vi "GeoData.vi"() -> ()   [LabVIEW 2017] (continued)
County\tH1\n71933\t5097\tBonnerdale\tAR\tMontgomery County\tH1\n71961\t5097\tOden\tAR\tMontgomery County\tH1\n71943\t5097\tGlenwood\tAR\tMontgomery County\tH1\n71969\t5097\tSims\tAR\tMontgomery County\tH1\n71965\t5097\tPencil bluff\tAR\tMontgomery County\tH1\n71970\t5097\tStory\tAR\tMontgomery County\tH1\n71960\t5097\tNorman\tAR\tMontgomery County\tH1\n71957\t5097\tMount ida\tAR\tMontgomery County\tH1\n71949\t5097\tJessieville\tAR\tMontgomery County\tH1\n71935\t5097\tCaddo gap\tAR\tMontgomery County\tH1\n71858\t5099\tRosston\tAR\tNevada County\tH1\n71764\t5099\tStephens\tAR\tNevada County\tH1\n71827\t5099\tBuckner\tAR\tNevada County\tH1\n71770\t5099\tWaldo\tAR\tNevada County\tH1\n71857\t5099\tPrescott\tAR\tNevada County\tH1\n71828\t5099\tCale\tAR\tNevada County\tH1\n71752\t5099\tMc neil\tAR\tNevada County\tH1\n71722\t5099\tBluff city\tAR\tNevada County\tH1\n71835\t5099\tEmmet\tAR\tNevada County\tH1\n71864\t5099\tWillisville\tAR\tNevada County\tH1\n71860\t5099\tStamps\tAR\tNevada County\tH1\n72628\t5101\tDeer\tAR\tNewton County\tH1\n72685\t5101\tWestern grove\tAR\tNewton County\tH1\n72641\t5101\tJasper\tAR\tNewton County\tH1\n72670\t5101\tPonca\tAR\tNewton County\tH1\n72601\t5101\tHarrison\tAR\tNewton County\tH1\n72624\t5101\tCompton\tAR\tNewton County\tH1\n72638\t5101\tGreen forest\tAR\tNewton County\tH1\n72683\t5101\tVendor\tAR\tNewton County\tH1\n72742\t5101\tKingston\tAR\tNewton County\tH1\n72666\t5101\tParthenon\tAR\tNewton County\tH1\n72640\t5101\tHasty\tAR\tNewton County\tH1\n72655\t5101\tMount judea\tAR\tNewton County\tH1\n72648\t5101\tMarble falls\tAR\tNewton County\tH1\n71701\t5103\tCamden\tAR\tOuachita County\tH1\n71764\t5103\tStephens\tAR\tOuachita County\tH1\n71720\t5103\tBearden\tAR\tOuachita County\tH1\n71763\t5103\tSparkman\tAR\tOuachita County\tH1\n71751\t5103\tLouann\tAR\tOuachita County\tH1\n71857\t5103\tPrescott\tAR\tOuachita County\tH1\n71762\t5103\tSmackover\tAR\tOuachita County\tH1\n71726\t5103\tChidester\tAR\tOuachita County\tH1\n72001\t5105\tAdona\tAR\tPerry County\tH1\n72857\t5105\tPlainview\tAR\tPerry County\tH1\n72126\t5105\tPerryville\tAR\tPerry County\tH1\n72135\t5105\tRoland\tAR\tPerry County\tH1\n72853\t5105\tOla\tAR\tPerry County\tH1\n72125\t5105\tPerry\tAR\tPerry County\tH1\n72034\t5105\tConway\tAR\tPerry County\tH1\n72025\t5105\tCasa\tAR\tPerry County\tH1\n72070\t5105\tHouston\tAR\tPerry County\tH1\n72016\t5105\tBigelow\tAR\tPerry County\tH1\n72366\t5107\tMarvell\tAR\tPhillips County\tH1\n72355\t5107\tLexa\tAR\tPhillips County\tH1\n72312\t5107\tBarton\tAR\tPhillips County\tH1\n72328\t5107\tCrumrod\tAR\tPhillips County\tH1\n72383\t5107\tTurner\tAR\tPhillips County\tH1\n72353\t5107\tLambrook\tAR\tPhillips County\tH1\n72342\t5107\tHelena\tAR\tPhillips County\tH1\n72374\t5107\tPoplar grove\tAR\tPhillips County\tH1\n72389\t5107\tWabash\tAR\tPhillips County\tH1\n72390\t5107\tWest helena\tAR\tPhillips County\tH1\n72369\t5107\tOneida\tAR\tPhillips County\tH1\n72333\t5107\tElaine\tAR\tPhillips County\tH1\n72367\t5107\tMellwood\tAR\tPhillips County\tH1\n72069\t5107\tHolly grove\tAR\tPhillips County\tH1\n71971\t5109\tUmpire\tAR\tPike County\tH1\n71943\t5109\tGlenwood\tAR\tPike County\tH1\n71922\t5109\tAntoine\tAR\tPike County\tH1\n71921\t5109\tAmity\tAR\tPike County\tH1\n71958\t5109\tMurfreesboro\tAR\tPike County\tH1\n71959\t5109\tNewhope\tAR\tPike County\tH1\n71952\t5109\tLangley\tAR\tPike County\tH1\n71852\t5109\tNashville\tAR\tPike County\tH1\n71935\t5109\tCaddo gap\tAR\tPike County\tH1\n71940\t5109\tDelight\tAR\tPike County\tH1\n71950\t5109\tKirby\tAR\tPike County\tH1\n72421\t5111\tCash\tAR\tPoinsett County\tH1\n72429\t5111\tFisher\tAR\tPoinsett County\tH1\n72475\t5111\tWaldenburg\tAR\tPoinsett County\tH1\n72472\t5111\tTrumann\tAR\tPoinsett County\tH1\n72354\t5111\tLepanto\tAR\tPoinsett County\tH1\n72432\t5111\tHarrisburg\tAR\tPoinsett County\tH1\n72386\t5111\tTyronza\tAR\tPoinsett County\tH1\n72419\t5111\tCaraway\tAR\tPoinsett County\tH1\n72365\t5111\tMarked tree\tAR\tPoinsett County\tH1\n72324\t5111\tCherry valley\tAR\tPoinsett County\tH1\n72377\t5111\tRivervale\tAR\tPoinsett County\tH1\n72479\t5111\tWeiner\tAR\tPoinsett County\tH1\n71944\t5113\tGrannis\tAR\tPolk County\tH1\n71945\t5113\tHatfield\tAR\tPolk County\tH1\n71961\t5113\tOden\tAR\tPolk County\tH1\n71937\t5113\tCove\tAR\tPolk County\tH1\n71841\t5113\tGillham\tAR\tPolk County\tH1\n71953\t5113\tMena\tAR\tPolk County\tH1\n71973\t5113\tWickes\tAR\tPolk County\tH1\n71972\t5113\tVandervoort\tAR\tPolk County\tH1\n71932\t5113\tBoard camp\tAR\tPolk County\tH1\n72801\t5115\tRussellville\tAR\tPope County\tH1\n72686\t5115\tWitts springs\tAR\tPope County\tH1\n72856\t5115\tPelsor\tAR\tPope County\tH1\n72802\t5115\tRussellville\tAR\tPope County\tH1\n72823\t5115\tAtkins\tAR\tPope County\tH1\n72843\t5115\tHector\tAR\tPope County\tH1\n72858\t5115\tPottsville\tAR\tPope County\tH1\n72847\t5115\tLondon\tAR\tPope County\tH1\n72811\t5115\tRussellville\tAR\tPope County\tH1\n72080\t5115\tJerusalem\tAR\tPope County\tH1\n72063\t5115\tHattieville\tAR\tPope County\tH1\n72846\t5115\tLamar\tAR\tPope County\tH1\n72837\t5115\tDover\tAR\tPope County\tH1\n72812\t5115\tRussellville\tAR\tPope County\tH1\n72679\t5115\tTilly\tAR\tPope County\tH1\n72170\t5117\tUlm\tAR\tPrairie County\tH1\n72134\t5117\tRoe\tAR\tPrairie County\tH1\n72086\t5117\tLonoke\tAR\tPrairie County\tH1\n72041\t5117\tDe valls bluff\tAR\tPrairie County\tH1\n72066\t5117\tHickory plains\tAR\tPrairie County\tH1\n72040\t5117\tDes arc\tAR\tPrairie County\tH1\n72060\t5117\tGriffithville\tAR\tPrairie County\tH1\n72160\t5117\tStuttgart\tAR\tPrairie County\tH1\n72024\t5117\tCarlisle\tAR\tPrairie County\tH1\n72017\t5117\tBiscoe\tAR\tPrairie County\tH1\n72176\t5117\tWard\tAR\tPrairie County\tH1\n72064\t5117\tHazen\tAR\tPrairie County\tH1\n72116\t5119\tNorth little rock\tAR\tPulaski County\tH1\n72205\t5119\tLittle rock\tAR\tPulaski County\tH1\n72223\t5119\tLittle rock\tAR\tPulaski County\tH1\n72204\t5119\tLittle rock\tAR\tPulaski County\tH1\n72207\t5119\tLittle rock\tAR\tPulaski County\tH1\n72227\t5119\tLittle rock\tAR\tPulaski County\tH1\n72078\t5119\tJacksonville\tAR\tPulaski County\tH1\n72199\t5119\tNorth little rock\tAR\tPulaski County\tH1\n72065\t5119\tHensley\tAR\tPulaski County\tH1\n72002\t5119\tAlexander\tAR\tPulaski County\tH1\n72209\t5119\tLittle rock\tAR\tPulaski County\tH1\n72126\t5119\tPerryville\tAR\tPulaski County\tH1\n72115\t5119\tNorth little rock\tAR\tPulaski County\tH1\n72255\t5119\tLittle rock\tAR\tPulaski County\tH1\n72023\t5119\tCabot\tAR\tPulaski County\tH1\n72120\t5119\tSherwood\tAR\tPulaski County\tH1\n72135\t5119\tRoland\tAR\tPulaski County\tH1\n72217\t5119\tLittle rock\tAR\tPulaski County\tH1\n72099\t5119\tLittle rock air force base\tAR\tPulaski County\tH1\n72046\t5119\tEngland\tAR\tPulaski County\tH1\n72113\t5119\tMaumelle\tAR\tPulaski County\tH1\n72202\t5119\tLittle rock\tAR\tPulaski County\tH1\n72214\t5119\tLittle rock\tAR\tPulaski County\tH1\n72117\t5119\tNorth little rock\tAR\tPulaski County\tH1\n72142\t5119\tScott\tAR\tPulaski County\tH1\n72190\t5119\tNorth little rock\tAR\tPulaski County\tH1\n72106\t5119\tMayflower\tAR\tPulaski County\tH1\n72053\t5119\tCollege station\tAR\tPulaski County\tH1\n72076\t5119\tJacksonville\tAR\tPulaski County\tH1\n72210\t5119\tLittle rock\tAR\tPulaski County\tH1\n72211\t5119\tLittle rock\tAR\tPulaski County\tH1\n72206\t5119\tLittle rock\tAR\tPulaski County\tH1\n72216\t5119\tLittle rock\tAR\tPulaski County\tH1\n72225\t5119\tLittle rock\tAR\tPulaski County\tH1\n72124\t5119\tNorth little rock\tAR\tPulaski County\tH1\n72173\t5119\tVilonia\tAR\tPulaski County\tH1\n72215\t5119\tLittle rock\tAR\tPulaski County\tH1\n72203\t5119\tLittle rock\tAR\tPulaski County\tH1\n72219\t5119\tLittle rock\tAR\tPulaski County\tH1\n72260\t5119\tLittle rock\tAR\tPulaski County\tH1\n72103\t5119\tMabelvale\tAR\tPulaski County\tH1\n72016\t5119\tBigelow\tAR\tPulaski County\tH1\n72132\t5119\tRedfield\tAR\tPulaski County\tH1\n72222\t5119\tLittle rock\tAR\tPulaski County\tH1\n72119\t5119\tNorth little rock\tAR\tPulaski County\tH1\n72180\t5119\tWoodson\tAR\tPulaski County\tH1\n72114\t5119\tNorth little rock\tAR\tPulaski County\tH1\n72201\t5119\tLittle rock\tAR\tPulaski County\tH1\n72212\t5119\tLittle rock\tAR\tPulaski County\tH1\n72118\t5119\tNorth little rock\tAR\tPulaski County\tH1\n72122\t5119\tParon\tAR\tPulaski County\tH1\n72221\t5119\tLittle rock\tAR\tPulaski County\tH1\n72231\t5119\tLittle rock\tAR\tPulaski County\tH1\n72183\t5119\tWrightsville\tAR\tPulaski County\tH1\n72164\t5119\tSweet home\tAR\tPulaski County\tH1\n72413\t5121\tBiggers\tAR\tRandolph County\tH1\n72449\t5121\tO kean\tAR\tRandolph County\tH1\n72455\t5121\tPocahontas\tAR\tRandolph County\tH1\n72554\t5121\tMammoth spring\tAR\tRandolph County\tH1\n72459\t5121\tRavenden\tAR\tRandolph County\tH1\n72462\t5121\tReyno\tAR\tRandolph County\tH1\n72476\t5121\tWalnut ridge\tAR\tRandolph County\tH1\n72460\t5121\tRavenden springs\tAR\tRandolph County\tH1\n72434\t5121\tImboden\tAR\tRandolph County\tH1\n72444\t5121\tMaynard\tAR\tRandolph County\tH1\n72478\t5121\tWarm springs\tAR\tRandolph County\tH1\n72422\t5121\tCorning\tAR\tRandolph County\tH1\n72425\t5121\tDelaplaine\tAR\tRandolph County\tH1\n72021\t5123\tBrinkley\tAR\tSt. Francis County\tH1\n72396\t5123\tWynne\tAR\tSt. Francis County\tH1\n72360\t5123\tMarianna\tAR\tSt. Francis County\tH1\n72346\t5123\tHeth\tAR\tSt. Francis County\tH1\n72392\t5123\tWheatley\tAR\tSt. Francis County\tH1\n72335\t5123\tForrest city\tAR\tSt. Francis County\tH1\n72348\t5123\tHughes\tAR\tSt. Francis County\tH1\n72326\t5123\tColt\tAR\tSt. Francis County\tH1\n72340\t5123\tGoodwin\tAR\tSt. Francis County\tH1\n72376\t5123\tProctor\tAR\tSt. Francis County\tH1\n72394\t5123\tWidener\tAR\tSt. Francis County\tH1\n72372\t5123\tPalestine\tAR\tSt. Francis County\tH1\n72359\t5123\tMadison\tAR\tSt. Francis County\tH1\n72322\t5123\tCaldwell\tAR\tSt. Francis County\tH1\n72019\t5125\tBenton\tAR\tSaline County\tH1\n72018\t5125\tBenton\tAR\tSaline County\tH1\n72065\t5125\tHensley\tAR\tSaline County\tH1\n72002\t5125\tAlexander\tAR\tSaline County\tH1\n72104\t5125\tMalvern\tAR\tSaline County\tH1\n72167\t5125\tTraskwood\tAR\tSaline County\tH1\n72022\t5125\tBryant\tAR\tSaline County\tH1\n72210\t5125\tLittle rock\tAR\tSaline County\tH1\n72206\t5125\tLittle rock\tAR\tSaline County\tH1\n72089\t5125\tBryant\tAR\tSaline County\tH1\n71909\t5125\tHot springs village\tAR\tSaline County\tH1\n72087\t5125\tLonsdale\tAR\tSaline County\tH1\n72015\t5125\tBenton\tAR\tSaline County\tH1\n72103\t5125\tMabelvale\tAR\tSaline County\tH1\n72011\t5125\tBauxite\tAR\tSaline County\tH1\n72122\t5125\tParon\tAR\tSaline County\tH1\n72944\t5127\tMansfield\tAR\tScott County\tH1\n72950\t5127\tParks\tAR\tScott County\tH1\n71953\t5127\tMena\tAR\tScott County\tH1\n72927\t5127\tBooneville\tAR\tScott County\tH1\n72841\t5127\tHarvey\tAR\tScott County\tH1\n72958\t5127\tWaldron\tAR\tScott County\tH1\n72926\t5127\tBoles\tAR\tScott County\tH1\n72838\t5127\tGravelly\tAR\tScott County\tH1\n72833\t5127\tDanville\tAR\tScott County\tH1\n72686\t5129\tWitts springs\tAR\tSearcy County\tH1\n72617\t5129\tBig flat\tAR\tSearcy County\tH1\n72636\t5129\tGilbert\tAR\tSearcy County\tH1\n72680\t5129\tTimbo\tAR\tSearcy County\tH1\n72685\t5129\tWestern grove\tAR\tSearcy County\tH1\n72650\t5129\tMarshall\tAR\tSearcy County\tH1\n72639\t5129\tHarriet\tAR\tSearcy County\tH1\n72629\t5129\tDennard\tAR\tSearcy County\tH1\n72675\t5129\tSaint joe\tAR\tSearcy County\tH1\n72633\t5129\tEverton\tAR\tSearcy County\tH1\n72645\t5129\tLeslie\tAR\tSearcy County\tH1\n72669\t5129\tPindall\tAR\tSearcy County\tH1\n72687\t5129\tYellville\tAR\tSearcy County\tH1\n72679\t5129\tTilly\tAR\tSearcy County\tH1\n72903\t5131\tFort smith\tAR\tSebastian County\tH1\n72933\t5131\tCharleston\tAR\tSebastian County\tH1\n72944\t5131\tMansfield\tAR\tSebastian County\tH1\n72918\t5131\tFort smith\tAR\tSebastian County\tH1\n72919\t5131\tFort smith\tAR\tSebastian County\tH1\n72936\t5131\tGreenwood\tAR\tSebastian County\tH1\n72916\t5131\tFort smith\tAR\tSebastian County\tH1\n72905\t5131\tFort smith\tAR\tSebastian County\tH1\n72904\t5131\tFort smith\tAR\tSebastian County\tH1\n72927\t5131\tBooneville\tAR\tSebastian County\tH1\n72938\t5131\tHartford\tAR\tSebastian County\tH1\n72940\t5131\tHuntington\tAR\tSebastian County\tH1\n72941\t5131\tLavaca\tAR\tSebastian County\tH1\n72908\t5131\tFort smith\tAR\tSebastian County\tH1\n72930\t5131\tCecil\tAR\tSebastian County\tH1\n72914\t5131\tFort smith\tAR\tSebastian County\tH1\n72913\t5131\tFort smith\tAR\tSebastian County\tH1\n72923\t5131\tBarling\tAR\tSebastian County\tH1\n72937\t5131\tHackett\tAR\tSebastian County\tH1\n72902\t5131\tFort smith\tAR\tSebastian County\tH1\n72917\t5131\tFort smith\tAR\tSebastian County\tH1\n72945\t5131\tMidland\tAR\tSebastian County\tH1\n72901\t5131\tFort smith\tAR\tSebastian County\tH1\n72906\t5131\tFort smith\tAR\tSebastian County\tH1\n71832\t5133\tDe queen\tAR\tSevier County\tH1\n71841\t5133\tGillham\tAR\tSevier County\tH1\n71833\t5133\tDierks\tAR\tSevier County\tH1\n71842\t5133\tHoratio\tAR\tSevier County\tH1\n71846\t5133\tLockesburg\tAR\tSevier County\tH1\n71823\t5133\tBen lomond\tAR\tSevier County\tH1\n72542\t5135\tHardy\tAR\tSharp County\tH1\n72469\t5135\tStrawberry\tAR\tSharp County\tH1\n72466\t5135\tSmithville\tAR\tSharp County\tH1\n72554\t5135\tMammoth spring\tAR\tSharp County\tH1\n72521\t5135\tCave city\tAR\tSharp County\tH1\n72529\t5135\tCherokee village\tAR\tSharp County\tH1\n72459\t5135\tRavenden\tAR\tSharp County\tH1\n72532\t5135\tEvening shade\tAR\tSharp County\tH1\n72579\t5135\tSulphur rock\tAR\tSharp County\tH1\n72482\t5135\tWilliford\tAR\tSharp County\tH1\n72513\t5135\tAsh flat\tAR\tSharp County\tH1\n72569\t5135\tPoughkeepsie\tAR\tSharp County\tH1\n72577\t5135\tSidney\tAR\tSharp County\tH1\n72153\t5137\tShirley\tAR\tStone County\tH1\n72044\t5137\tEdgemont\tAR\tStone County\tH1\n72051\t5137\tFox\tAR\tStone County\tH1\n72617\t5137\tBig flat\tAR\tStone County\tH1\n72567\t5137\tPleasant grove\tAR\tStone County\tH1\n72680\t5137\tTimbo\tAR\tStone County\tH1\n72556\t5137\tMelbourne\tAR\tStone County\tH1\n72530\t5137\tDrasco\tAR\tStone County\tH1\n72650\t5137\tMarshall\tAR\tStone County\tH1\n72550\t5137\tLocust grove\tAR\tStone County\tH1\n72540\t5137\tGuion\tAR\tStone County\tH1\n72555\t5137\tMarcella\tAR\tStone County\tH1\n72645\t5137\tLeslie\tAR\tStone County\tH1\n72657\t5137\tTimbo\tAR\tStone County\tH1\n72031\t5137\tClinton\tAR\tStone County\tH1\n72519\t5137\tCalico rock\tAR\tStone County\tH1\n72533\t5137\tFifty six\tAR\tStone County\tH1\n72560\t5137\tMountain view\tAR\tStone County\tH1\n72663\t5137\tOnia\tAR\tStone County\tH1\n71730\t5139\tEl dorado\tAR\tUnion County\tH1\n71747\t5139\tHuttig\tAR\tUnion County\tH1\n71750\t5139\tLawson\tAR\tUnion County\tH1\n71764\t5139\tStephens\tAR\tUnion County\tH1\n71759\t5139\tNorphlet\tAR\tUnion County\tH1\n71753\t5139\tMagnolia\tAR\tUnion County\tH1\n71762\t5139\tSmackover\tAR\tUnion County\tH1\n71731\t5139\tEl dorado\tAR\tUnion County\tH1\n71724\t5139\tCalion\tAR\tUnion County\tH1\n71765\t5139\tStrong\tAR\tUnion County\tH1\n71749\t5139\tJunction city\tAR\tUnion County\tH1\n71758\t5139\tMount holly\tAR\tUnion County\tH1\n72013\t5141\tBee branch\tAR\tVan Buren County\tH1\n72153\t5141\tShirley\tAR\tVan Buren County\tH1\n72039\t5141\tDamascus\tAR\tVan Buren County\tH1\n72030\t5141\tCleveland\tAR\tVan Buren County\tH1\n72067\t5141\tHigden\tAR\tVan Buren County\tH1\n72131\t5141\tQuitman\tAR\tVan Buren County\tH1\n72028\t5141\tChoctaw\tAR\tVan Buren County\tH1\n72629\t5141\tDennard\tAR\tVan Buren County\tH1\n72080\t5141\tJerusalem\tAR\tVan Buren County\tH1\n72645\t5141\tLeslie\tAR\tVan Buren County\tH1\n72031\t5141\tClinton\tAR\tVan Buren County\tH1\n72088\t5141\tFairfield bay\tAR\tVan Buren County\tH1\n72141\t5141\tScotland\tAR\tVan Buren County\tH1\n72679\t5141\tTilly\tAR\tVan Buren County\tH1\n72703\t5143\tFayetteville\tAR\tWashington County\tH1\n72730\t5143\tFarmington\tAR\tWashington County\tH1\n72773\t5143\tWesley\tAR\tWashington County\tH1\n72765\t5143\tSpringdale\tAR\tWashington County\tH1\n72728\t5143\tElm springs\tAR\tWashington County\tH1\n72761\t5143\tSiloam springs\tAR\tWashington County\tH1\n72764\t5143\tSpringdale\tAR\tWashington County\tH1\n72741\t5143\tJohnson\tAR\tWashington County\tH1\n72770\t5143\tTontitown\tAR\tWashington County\tH1\n72717\t5143\tCanehill\tAR\tWashington County\tH1\n72734\t5143\tGentry\tAR\tWashington County\tH1\n72727\t5143\tElkins\tAR\tWashington County\tH1\n72769\t5143\tSummers\tAR\tWashington County\tH1\n72766\t5143\tSpringdale\tAR\tWashington County\tH1\n72749\t5143\tMorrow\tAR\tWashington County\tH1\n72704\t5143\tFayetteville\tAR\tWashington County\tH1\n72959\t5143\tWinslow\tAR\tWashington County\tH1\n72948\t5143\tNatural dam\tAR\tWashington County\tH1\n72737\t5143\tGreenland\tAR\tWashington County\tH1\n72738\t5143\tHindsville\tAR\tWashington County\tH1\n72729\t5143\tEvansville\tAR\tWashington County\tH1\n72762\t5143\tSpringdale\tAR\tWashington County\tH1\n72774\t5143\tWest fork\tAR\tWashington County\tH1\n72753\t5143\tPrairie grove\tAR\tWashington County\tH1\n72702\t5143\tFayetteville\tAR\tWashington County\tH1\n72744\t5143\tLincoln\tAR\tWashington County\tH1\n72735\t5143\tGoshen\tAR\tWashington County\tH1\n72701\t5143\tFayetteville\tAR\tWashington County\tH1\n72010\t5145\tBald knob\tAR\tWhite County\tH1\n72568\t5145\tPleasant plains\tAR\tWhite County\tH1\n72068\t5145\tHigginson\tAR\tWhite County\tH1\n72178\t5145\tWest point\tAR\tWhite County\tH1\n72139\t5145\tRussell\tAR\tWhite County\tH1\n72012\t5145\tBeebe\tAR\tWhite County\tH1\n72121\t5145\tPangburn\tAR\tWhite County\tH1\n72085\t5145\tLetona\tAR\tWhite County\tH1\n72081\t5145\tJudsonia\tAR\tWhite County\tH1\n72102\t5145\tMc rae\tAR\tWhite County\tH1\n72143\t5145\tSearcy\tAR\tWhite County\tH1\n72052\t5145\tGarner\tAR\tWhite County\tH1\n72082\t5145\tKensett\tAR\tWhite County\tH1\n72045\t5145\tEl paso\tAR\tWhite County\tH1\n72060\t5145\tGriffithville\tAR\tWhite County\tH1\n72149\t5145\tSearcy\tAR\tWhite County\tH1\n72020\t5145\tBradford\tAR\tWhite County\tH1\n72173\t5145\tVilonia\tAR\tWhite County\tH1\n72111\t5145\tMount vernon\tAR\tWhite County\tH1\n72145\t5145\tSearcy\tAR\tWhite County\tH1\n72136\t5145\tRomance\tAR\tWhite County\tH1\n72137\t5145\tRose bud\tAR\tWhite County\tH1\n72112\t5147\tNewport\tAR\tWoodruff County\tH1\n72021\t5147\tBrinkley\tAR\tWoodruff County\tH1\n72396\t5147\tWynne\tAR\tWoodruff County\tH1\n72006\t5147\tAugusta\tAR\tWoodruff County\tH1\n72123\t5147\tPatterson\tAR\tWoodruff County\tH1\n72392\t5147\tWheatley\tAR\tWoodruff County\tH1\n72059\t5147\tGregory\tAR\tWoodruff County\tH1\n72101\t5147\tMc crory\tAR\tWoodruff County\tH1\n72036\t5147\tCotton plant\tAR\tWoodruff County\tH1\n72074\t5147\tHunter\tAR\tWoodruff County\tH1\n72857\t5149\tPlainview\tAR\tYell County\tH1\n72943\t5149\tMagazine\tAR\tYell County\tH1\n72853\t5149\tOla\tAR\tYell County\tH1\n72842\t5149\tHavana\tAR\tYell County\tH1\n72824\t5149\tBelleville\tAR\tYell County\tH1\n72828\t5149\tBriggsville\tAR\tYell County\tH1\n72841\t5149\tHarvey\tAR\tYell County\tH1\n72025\t5149\tCasa\tAR\tYell County\tH1\n72827\t5149\tBluffton\tAR\tYell County\tH1\n72860\t5149\tRover\tAR\tYell County\tH1\n72829\t5149\tCenterville\tAR\tYell County\tH1\n72834\t5149\tDardanelle\tAR\tYell County\tH1\n72838\t5149\tGravelly\tAR\tYell County\tH1\n72833\t5149\tDanville\tAR\tYell County\tH1\n94501\t6001\tAlameda\tCA\tAlameda County\tH1\n94560\t6001\tNewark\tCA\tAlameda County\tH1\n94577\t6001\tSan leandro\tCA\tAlameda County\tH1\n94578\t6001\tSan leandro\tCA\tAlameda County\tH1\n94550\t6001\tLivermore\tCA\tAlameda County\tH1\n94611\t6001\tOakland\tCA\tAlameda County\tH1\n94705\t6001\tBerkeley\tCA\tAlameda County\tH1\n94505\t6001\tDiscovery bay\tCA\tAlameda County\tH1\n94568\t6001\tDublin\tCA\tAlameda County\tH1\n94551\t6001\tLivermore\tCA\tAlameda County\tH1\n94586\t6001\tSunol\tCA\tAlameda County\tH1\n94702\t6001\tBerkeley\tCA\tAlameda County\tH1\n94709\t6001\tBerkeley\tCA\tAlameda County\tH1\n94662\t6001\tEmeryville\tCA\tAlameda County\tH1\n94514\t6001\tByron\tCA\tAlameda County\tH1\n94544\t6001\tHayward\tCA\tAlameda County\tH1\n94566\t6001\tPleasanton\tCA\tAlameda County\tH1\n94608\t6001\tEmeryville\tCA\tAlameda County\tH1\n94609\t6001\tOakland\tCA\tAlameda County\tH1\n94707\t6001\tBerkeley\tCA\tAlameda County\tH1\n94604\t6001\tOakland\tCA\tAlameda County\tH1\n95035\t6001\tMilpitas\tCA\tAlameda County\tH1\n94543\t6001\tHayward\tCA\tAlameda County\tH1\n94614\t6001\tOakland\tCA\tAlameda County\tH1\n94712\t6001\tBerkeley\tCA\tAlameda County\tH1\n94540\t6001\tHayward\tCA\tAlameda County\tH1\n94541\t6001\tHayward\tCA\tAlameda County\tH1\n94555\t6001\tFremont\tCA\tAlameda County\tH1\n94579\t6001\tSan leandro\tCA\tAlameda County\tH1\n94612\t6001\tOakland\tCA\tAlameda County\tH1\n94601\t6001\tOakland\tCA\tAlameda County\tH1\n94623\t6001\tOakland\tCA\tAlameda County\tH1\n94536\t6001\tFremont\tCA\tAlameda County\tH1\n94552\t6001\tCastro valley\tCA\tAlameda County\tH1\n94621\t6001\tOakland\tCA\tAlameda County\tH1\n94703\t6001\tBerkeley\tCA\tAlameda County\tH1\n95377\t6001\tTracy\tCA\tAlameda County\tH1\n94708\t6001\tBerkeley\tCA\tAlameda County\tH1\n94620\t6001\tPiedmont\tCA\tAlameda County\tH1\n94615\t6001\tOakland\tCA\tAlameda County\tH1\n94546\t6001\tCastro valley\tCA\tAlameda County\tH1\n94588\t6001\tPleasanton\tCA\tAlameda County\tH1\n94603\t6001\tOakland\tCA\tAlameda County\tH1\n94605\t6001\tOakland\tCA\tAlameda County\tH1\n94606\t6001\tOakland\tCA\tAlameda County\tH1\n94704\t6001\tBerkeley\tCA\tAlameda County\tH1\n94619\t6001\tOakland\tCA\tAlameda County\tH1\n94706\t6001\tAlbany\tCA\tAlameda County\tH1\n94557\t6001\tHayward\tCA\tAlameda County\tH1\n94539\t6001\tFremont\tCA\tAlameda County\tH1\n94542\t6001\tHayward\tCA\tAlameda County\tH1\n94587\t6001\tUnion city\tCA\tAlameda County\tH1\n94545\t6001\tHayward\tCA\tAlameda County\tH1\n94607\t6001\tOakland\tCA\tAlameda County\tH1\n94618\t6001\tOakland\tCA\tAlameda County\tH1\n94602\t6001\tOakland\tCA\tAlameda County\tH1\n94720\t6001\tBerkeley\tCA\tAlameda County\tH1\n95391\t6001\tTracy\tCA\tAlameda County\tH1\n94701\t6001\tBerkeley\tCA\tAlameda County\tH1\n94661\t6001\tOakland\tCA\tAlameda County\tH1\n94613\t6001\tOakland\tCA\tAlameda County\tH1\n94502\t6001\tAlameda\tCA\tAlameda County\tH1\n94538\t6001\tFremont\tCA\tAlameda County\tH1\n94580\t6001\tSan lorenzo\tCA\tAlameda County\tH1\n94610\t6001\tOakland\tCA\tAlameda County\tH1\n94710\t6001\tBerkeley\tCA\tAlameda County\tH1\n94537\t6001\tFremont\tCA\tAlameda County\tH1\n94624\t6001\tOakland\tCA\tAlameda County\tH1\n94666\t6001\tOakland\tCA\tAlameda County\tH1\n96120\t6003\tMarkleeville\tCA\tAlpine County\tH1\n95223\t6003\tArnold\tCA\tAlpine County\tH1\n95666\t6005\tPioneer\tCA\tAmador County\tH1\n95675\t6005\tRiver pines\tCA\tAmador County\tH1\n95669\t6005\tPlymouth\tCA\tAmador County\tH1\n95699\t6005\tDrytown\tCA\tAmador County\tH1\n95646\t6005\tKirkwood\tCA\tAmador County\tH1\n95640\t6005\tIone\tCA\tAmador County\tH1\n95629\t6005\tFiddletown\tCA\tAmador County\tH1\n95689\t6005\tVolcano\tCA\tAmador County\tH1\n95685\t6005\tSutter creek\tCA\tAmador County\tH1\n95654\t6005\tMartell\tCA\tAmador County\tH1\n95665\t6005\tPine grove\tCA\tAmador County\tH1\n95601\t6005\tAmador city\tCA\tAmador County\tH1\n95642\t6005\tJackson\tCA\tAmador County\tH1\n95917\t6007\tBiggs\tCA\tButte County\tH1\n95940\t6007\tFeather falls\tCA\tButte County\tH1\n95929\t6007\tChico\tCA\tButte County\tH1\n95954\t6007\tMagalia\tCA\tButte County\tH1\n95926\t6007\tChico\tCA\tButte County\tH1\n95901\t6007\tMarysville\tCA\tButte County\tH1\n95973\t6007\tChico\tCA\tButte County\tH1\n95914\t6007\tBangor\tCA\tButte County\tH1\n95948\t6007\tGridley\tCA\tButte County\tH1\n95927\t6007\tChico\tCA\tButte County\tH1\n95942\t6007\tForest ranch\tCA\tButte County\tH1\n95967\t6007\tParadise\tCA\tButte County\tH1\n95968\t6007\tPalermo\tCA\tButte County\tH1\n95958\t6007\tNelson\tCA\tButte County\tH1\n95974\t6007\tRichvale\tCA\tButte County\tH1\n95916\t6007\tBerry creek\tCA\tButte County\tH1\n95930\t6007\tClipper mills\tCA\tButte County\tH1\n95969\t6007\tParadise\tCA\tButte County\tH1\n95938\t6007\tDurham\tCA\tButte County\tH1\n95941\t6007\tForbestown\tCA\tButte County\tH1\n95976\t6007\tChico\tCA\tButte County\tH1\n95965\t6007\tOroville\tCA\tButte County\tH1\n95978\t6007\tStirling city\tCA\tButte County\tH1\n95928\t6007\tChico\tCA\tButte County\tH1\n95966\t6007\tOroville\tCA\tButte County\tH1\n95228\t6009\tCopperopolis\tCA\tCalaveras County\tH1\n95246\t6009\tMountain ranch\tCA\tCalaveras County\tH1\n95255\t6009\tWest point\tCA\tCalaveras County\tH1\n95251\t6009\tVallecito\tCA\tCalaveras County\tH1\n95248\t6009\tRail road flat\tCA\tCalaveras County\tH1\n95229\t6009\tDouglas flat\tCA\tCalaveras County\tH1\n95223\t6009\tArnold\tCA\tCalaveras County\tH1\n95221\t6009\tAltaville\tCA\tCalaveras County\tH1\n95226\t6009\tCampo seco\tCA\tCalaveras County\tH1\n95222\t6009\tAngels camp\tCA\tCalaveras County\tH1\n95232\t6009\tGlencoe\tCA\tCalaveras County\tH1\n95249\t6009\tSan andreas\tCA\tCalaveras County\tH1\n95233\t6009\tHathaway pines\tCA\tCalaveras County\tH1\n95225\t6009\tBurson\tCA\tCalaveras County\tH1\n95252\t6009\tValley springs\tCA\tCalaveras County\tH1\n95247\t6009\tMurphys\tCA\tCalaveras County\tH1\n95245\t6009\tMokelumne hill\tCA\tCalaveras County\tH1\n95254\t6009\tWallace\tCA\tCalaveras County\tH1\n95224\t6009\tAvery\tCA\tCalaveras County\tH1\n95236\t6009\tLinden\tCA\tCalaveras County\tH1\n95230\t6009\tFarmington\tCA\tCalaveras County\tH1\n95257\t6009\tWilseyville\tCA\tCalaveras County\tH1\n95645\t6011\tKnights landing\tCA\tColusa County\tH1\n95955\t6011\tMaxwell\tCA\tColusa County\tH1\n95988\t6011\tWillows\tCA\tColusa County\tH1\n95957\t6011\tMeridian\tCA\tColusa County\tH1\n95970\t6011\tPrinceton\tCA\tColusa County\tH1\n95979\t6011\tStonyford\tCA\tColusa County\tH1\n95939\t6011\tElk creek\tCA\tColusa County\tH1\n95950\t6011\tGrimes\tCA\tColusa County\tH1\n95912\t6011\tArbuckle\tCA\tColusa County\tH1\n95932\t6011\tColusa\tCA\tColusa County\tH1\n95987\t6011\tWilliams\tCA\tColusa County\tH1\n94509\t6013\tAntioch\tCA\tContra Costa County\tH1\n94519\t6013\tConcord\tCA\tContra Costa County\tH1\n94553\t6013\tMartinez\tCA\tContra Costa County\tH1\n94561\t6013\tOakley\tCA\tContra Costa County\tH1\n94611\t6013\tOakland\tCA\tContra Costa County\tH1\n94598\t6013\tWalnut creek\tCA\tContra Costa County\tH1\n94524\t6013\tConcord\tCA\tContra Costa County\tH1\n94526\t6013\tDanville\tCA\tContra Costa County\tH1\n94505\t6013\tDiscovery bay\tCA\tContra Costa County\tH1\n94568\t6013\tDublin\tCA\tContra Costa County\tH1\n94551\t6013\tLivermore\tCA\tContra Costa County\tH1\n94582\t6013\tSan ramon\tCA\tContra Costa County\tH1\n94547\t6013\tHercules\tCA\tContra Costa County\tH1\n94522\t6013\tConcord\tCA\tContra Costa County\tH1\n94570\t6013\tMoraga\tCA\tContra Costa County\tH1\n94513\t6013\tBrentwood\tCA\tContra Costa County\tH1\n94514\t6013\tByron\tCA\tContra Costa County\tH1\n94525\t6013\tCrockett\tCA\tContra Costa County\tH1\n94565\t6013\tPittsburg\tCA\tContra Costa County\tH1\n94707\t6013\tBerkeley\tCA\tContra Costa County\tH1\n94804\t6013\tRichmond\tCA\tContra Costa County\tH1\n94850\t6013\tRichmond\tCA\tContra Costa County\tH1\n94549\t6013\tLafayette\tCA\tContra Costa County\tH1\n94805\t6013\tRichmond\tCA\tContra Costa County\tH1\n94806\t6013\tSan pablo\tCA\tContra Costa County\tH1\n94530\t6013\tEl cerrito\tCA\tContra Costa County\tH1\n94564\t6013\tPinole\tCA\tContra Costa County\tH1\n94583\t6013\tSan ramon\tCA\tContra Costa County\tH1\n94803\t6013\tEl sobrante\tCA\tContra Costa County\tH1\n94708\t6013\tBerkeley\tCA\tContra Costa County\tH1\n94575\t6013\tMoraga\tCA\tContra Costa County\tH1\n94518\t6013\tConcord\tCA\tContra Costa County\tH1\n94520\t6013\tConcord\tCA\tContra Costa County\tH1\n94521\t6013\tConcord\tCA\tContra Costa County\tH1\n94531\t6013\tAntioch\tCA\tContra Costa County\tH1\n94507\t6013\tAlamo\tCA\tContra Costa County\tH1\n94572\t6013\tRodeo\tCA\tContra Costa County\tH1\n94588\t6013\tPleasanton\tCA\tContra Costa County\tH1\n94596\t6013\tWalnut creek\tCA\tContra Costa County\tH1\n94706\t6013\tAlbany\tCA\tContra Costa County\tH1\n94511\t6013\tBethel island\tCA\tContra Costa County\tH1\n94516\t6013\tCanyon\tCA\tContra Costa County\tH1\n94569\t6013\tPort costa\tCA\tContra Costa County\tH1\n94517\t6013\tClayton\tCA\tContra Costa County\tH1\n94506\t6013\tDanville\tCA\tContra Costa County\tH1\n94563\t6013\tOrinda\tCA\tContra Costa County\tH1\n94801\t6013\tRichmond\tCA\tContra Costa County\tH1\n94802\t6013\tRichmond\tCA\tContra Costa County\tH1\n94820\t6013\tEl sobrante\tCA\tContra Costa County\tH1\n94807\t6013\tRichmond\tCA\tContra Costa County\tH1\n94523\t6013\tPleasant hill\tCA\tContra Costa County\tH1\n94556\t6013\tMoraga\tCA\tContra Costa County\tH1\n94595\t6013\tWalnut creek\tCA\tContra Costa County\tH1\n94597\t6013\tWalnut creek\tCA\tContra Costa County\tH1\n94548\t6013\tKnightsen\tCA\tContra Costa County\tH1\n94528\t6013\tDiablo\tCA\tContra Costa County\tH1\n95538\t6015\tFort dick\tCA\tDel Norte County\tH1\n95543\t6015\tGasquet\tCA\tDel Norte County\tH1\n95567\t6015\tSmith river\tCA\tDel Norte County\tH1\n95548\t6015\tKlamath\tCA\tDel Norte County\tH1\n95532\t6015\tCrescent city\tCA\tDel Norte County\tH1\n95531\t6015\tCrescent city\tCA\tDel Norte County\tH1\n95666\t6017\tPioneer\tCA\tEl Dorado County\tH1\n95656\t6017\tMount aukum\tCA\tEl Dorado County\tH1\n96155\t6017\tSouth lake tahoe\tCA\tEl Dorado County\tH1\n95634\t6017\tGeorgetown\tCA\tEl Dorado County\tH1\n95726\t6017\tPollock pines\tCA\tEl Dorado County\tH1\n96158\t6017\tSouth lake tahoe\tCA\tEl Dorado County\tH1\n95629\t6017\tFiddletown\tCA\tEl Dorado County\tH1\n95672\t6017\tRescue\tCA\tEl Dorado County\tH1\n95682\t6017\tShingle springs\tCA\tEl Dorado County\tH1\n95613\t6017\tColoma\tCA\tEl Dorado County\tH1\n95684\t6017\tSomerset\tCA\tEl Dorado County\tH1\n95720\t6017\tKyburz\tCA\tEl Dorado County\tH1\n96150\t6017\tSouth lake tahoe\tCA\tEl Dorado County\tH1\n95614\t6017\tCool\tCA\tEl Dorado County\tH1\n95667\t6017\tPlacerville\tCA\tEl Dorado County\tH1\n95635\t6017\tGreenwood\tCA\tEl Dorado County\tH1\n95636\t6017\tGrizzly flats\tCA\tEl Dorado County\tH1\n95623\t6017\tEl dorado\tCA\tEl Dorado County\tH1\n95619\t6017\tDiamond springs\tCA\tEl Dorado County\tH1\n95664\t6017\tPilot hill\tCA\tEl Dorado County\tH1\n95735\t6017\tTwin bridges\tCA\tEl Dorado County\tH1\n96151\t6017\tSouth lake tahoe\tCA\tEl Dorado County\tH1\n95762\t6017\tEl dorado hills\tCA\tEl Dorado County\tH1\n95709\t6017\tCamino\tCA\tEl Dorado County\tH1\n95633\t6017\tGarden valley\tCA\tEl Dorado County\tH1\n95651\t6017\tLotus\tCA\tEl Dorado County\tH1\n96142\t6017\tTahoma\tCA\tEl Dorado County\tH1\n95721\t6017\tEcho lake\tCA\tEl Dorado County\tH1\n93625\t6019\tFowler\tCA\tFresno County\tH1\n93619\t6019\tClovis\tCA\tFresno County\tH1\n93647\t6019\tOrosi\tCA\tFresno County\tH1\n93613\t6019\tClovis\tCA\tFresno County\tH1\n93776\t6019\tFresno\tCA\tFresno County\tH1\n93778\t6019\tFresno\tCA\tFresno County\tH1\n93707\t6019\tFresno\tCA\tFresno County\tH1\n93709\t6019\tFresno\tCA\tFresno County\tH1\n93720\t6019\tFresno\tCA\tFresno County\tH1\n93675\t6019\tSquaw valley\tCA\tFresno County\tH1\n93650\t6019\tFresno\tCA\tFresno County\tH1\n93664\t6019\tShaver lake\tCA\tFresno County\tH1\n93716\t6019\tFresno\tCA\tFresno County\tH1\n93777\t6019\tFresno\tCA\tFresno County\tH1\n93708\t6019\tFresno\tCA\tFresno County\tH1\n93741\t6019\tFresno\tCA\tFresno County\tH1\n93634\t6019\tLakeshore\tCA\tFresno County\tH1\n93761\t6019\tFresno\tCA\tFresno County\tH1\n93727\t6019\tFresno\tCA\tFresno County\tH1\n93611\t6019\tClovis\tCA\tFresno County\tH1\n93612\t6019\tClovis\tCA\tFresno County\tH1\n93609\t6019\tCaruthers\tCA\tFresno County\tH1\n93640\t6019\tMendota\tCA\tFresno County\tH1\n93641\t6019\tMiramonte\tCA\tFresno County\tH1\n93626\t6019\tFriant\tCA\tFresno County\tH1\n93628\t6019\tHume\tCA\tFresno County\tH1\n93711\t6019\tFresno\tCA\tFresno County\tH1\n93722\t6019\tFresno\tCA\tFresno County\tH1\n93701\t6019\tFresno\tCA\tFresno County\tH1\n93714\t6019\tFresno\tCA\tFresno County\tH1\n93794\t6019\tFresno\tCA\tFresno County\tH1\n93234\t6019\tHuron\tCA\tFresno County\tH1\n93718\t6019\tFresno\tCA\tFresno County\tH1\n93760\t6019\tFresno\tCA\tFresno County\tH1\n93786\t6019\tFresno\tCA\tFresno County\tH1\n93888\t6019\tFresno\tCA\tFresno County\tH1\n93744\t6019\tFresno\tCA\tFresno County\tH1\n93620\t6019\tDos palos\tCA\tFresno County\tH1\n93747\t6019\tFresno\tCA\tFresno County\tH1\n93603\t6019\tBadger\tCA\tFresno County\tH1\n93729\t6019\tFresno\tCA\tFresno County\tH1\n93621\t6019\tDunlap\tCA\tFresno County\tH1\n93654\t6019\tReedley\tCA\tFresno County\tH1\n93662\t6019\tSelma\tCA\tFresno County\tH1\n93702\t6019\tFresno\tCA\tFresno County\tH1\n93656\t6019\tRiverdale\tCA\tFresno County\tH1\n93657\t6019\tSanger\tCA\tFresno County\tH1\n93792\t6019\tFresno\tCA\tFresno County\tH1\n93740\t6019\tFresno\tCA\tFresno County\tH1\n93606\t6019\tBiola\tCA\tFresno County\tH1\n93764\t6019\tFresno\tCA\tFresno County\tH1\n93627\t6019\tHelm\tCA\tFresno County\tH1\n93704\t6019\tFresno\tCA\tFresno County\tH1\n93705\t6019\tFresno\tCA\tFresno County\tH1\n93726\t6019\tFresno\tCA\tFresno County\tH1\n93703\t6019\tFresno\tCA\tFresno County\tH1\n93710\t6019\tFresno\tCA\tFresno County\tH1\n93728\t6019\tFresno\tCA\tFresno County\tH1\n93630\t6019\tKerman\tCA\tFresno County\tH1\n93637\t6019\tMadera\tCA\tFresno County\tH1\n93772\t6019\tFresno\tCA\tFresno County\tH1\n93706\t6019\tFresno\tCA\tFresno County\tH1\n93616\t6019\tDel rey\tCA\tFresno County\tH1\n93715\t6019\tFresno\tCA\tFresno County\tH1\n93660\t6019\tSan joaquin\tCA\tFresno County\tH1\n93668\t6019\tTranquillity\tCA\tFresno County\tH1\n93712\t6019\tFresno\tCA\tFresno County\tH1\n93779\t6019\tFresno\tCA\tFresno County\tH1\n93725\t6019\tFresno\tCA\tFresno County\tH1\n93618\t6019\tDinuba\tCA\tFresno County\tH1\n93646\t6019\tOrange cove\tCA\tFresno County\tH1\n93648\t6019\tParlier\tCA\tFresno County\tH1\n93631\t6019\tKingsburg\tCA\tFresno County\tH1\n93773\t6019\tFresno\tCA\tFresno County\tH1\n93793\t6019\tFresno\tCA\tFresno County\tH1\n93844\t6019\tFresno\tCA\tFresno County\tH1\n93624\t6019\tFive points\tCA\tFresno County\tH1\n93642\t6019\tMono hot springs\tCA\tFresno County\tH1\n93723\t6019\tFresno\tCA\tFresno County\tH1\n93602\t6019\tAuberry\tCA\tFresno County\tH1\n93622\t6019\tFirebaugh\tCA\tFresno County\tH1\n93724\t6019\tFresno\tCA\tFresno County\tH1\n93771\t6019\tFresno\tCA\tFresno County\tH1\n93717\t6019\tFresno\tCA\tFresno County\tH1\n93775\t6019\tFresno\tCA\tFresno County\tH1\n93649\t6019\tPiedra\tCA\tFresno County\tH1\n93605\t6019\tBig creek\tCA\tFresno County\tH1\n93765\t6019\tFresno\tCA\tFresno County\tH1\n93210\t6019\tCoalinga\tCA\tFresno County\tH1\n93745\t6019\tFresno\tCA\tFresno County\tH1\n93608\t6019\tCantua creek\tCA\tFresno County\tH1\n93242\t6019\tLaton\tCA\tFresno County\tH1\n93730\t6019\tFresno\tCA\tFresno County\tH1\n93737\t6019\tFresno\tCA\tFresno County\tH1\n93755\t6019\tFresno\tCA\tFresno County\tH1\n93774\t6019\tFresno\tCA\tFresno County\tH1\n93721\t6019\tFresno\tCA\tFresno County\tH1\n93667\t6019\tTollhouse\tCA\tFresno County\tH1\n93651\t6019\tPrather\tCA\tFresno County\tH1\n93652\t6019\tRaisin city\tCA\tFresno County\tH1\n93791\t6019\tFresno\tCA\tFresno County\tH1\n93790\t6019\tFresno\tCA\tFresno County\tH1\n93750\t6019\tFresno\tCA\tFresno County\tH1\n95951\t6021\tHamilton city\tCA\tGlenn County\tH1\n95963\t6021\tOrland\tCA\tGlenn County\tH1\n95913\t6021\tArtois\tCA\tGlenn County\tH1\n95988\t6021\tWillows\tCA\tGlenn County\tH1\n95943\t6021\tGlenn\tCA\tGlenn County\tH1\n95970\t6021\tPrinceton\tCA\tGlenn County\tH1\n95939\t6021\tElk creek\tCA\tGlenn County\tH1\n95920\t6021\tButte city\tCA\tGlenn County\tH1\n95540\t6023\tFortuna\tCA\tHumboldt County\tH1\n95560\t6023\tRedway\tCA\tHumboldt County\tH1\n95550\t6023\tKorbel\tCA\tHumboldt County\tH1\n95563\t6023\tSalyer\tCA\tHumboldt County\tH1\n95501\t6023\tEureka\tCA\tHumboldt County\tH1\n95524\t6023\tBayside\tCA\tHumboldt County\tH1\n95528\t6023\tCarlotta\tCA\tHumboldt County\tH1\n95565\t6023\tScotia\tCA\tHumboldt County\tH1\n95518\t6023\tArcata\tCA\tHumboldt County\tH1\n95521\t6023\tArcata\tCA\tHumboldt County\tH1\n95570\t6023\tTrinidad\tCA\tHumboldt County\tH1\n95526\t6023\tBridgeville\tCA\tHumboldt County\tH1\n95546\t6023\tHoopa\tCA\tHumboldt County\tH1\n95589\t6023\tWhitethorn\tCA\tHumboldt County\tH1\n95564\t6023\tSamoa\tCA\tHumboldt County\tH1\n95547\t6023\tHydesville\tCA\tHumboldt County\tH1\n95559\t6023\tPhillipsville\tCA\tHumboldt County\tH1\n95542\t6023\tGarberville\tCA\tHumboldt County\tH1\n95551\t6023\tLoleta\tCA\tHumboldt County\tH1\n95514\t6023\tBlocksburg\tCA\tHumboldt County\tH1\n95503\t6023\tEureka\tCA\tHumboldt County\tH1\n95519\t6023\tMckinleyville\tCA\tHumboldt County\tH1\n95536\t6023\tFerndale\tCA\tHumboldt County\tH1\n95511\t6023\tAlderpoint\tCA\tHumboldt County\tH1\n95502\t6023\tEureka\tCA\tHumboldt County\tH1\n95555\t6023\tOrick\tCA\tHumboldt County\tH1\n95571\t6023\tWeott\tCA\tHumboldt County\tH1\n95545\t6023\tHoneydew\tCA\tHumboldt County\tH1\n95556\t6023\tOrleans\tCA\tHumboldt County\tH1\n95562\t6023\tRio dell\tCA\tHumboldt County\tH1\n95558\t6023\tPetrolia\tCA\tHumboldt County\tH1\n95549\t6023\tKneeland\tCA\tHumboldt County\tH1\n95587\t6023\tPiercy\tCA\tHumboldt County\tH1\n95573\t6023\tWillow creek\tCA\tHumboldt County\tH1\n95537\t6023\tFields landing\tCA\tHumboldt County\tH1\n95525\t6023\tBlue lake\tCA\tHumboldt County\tH1\n95554\t6023\tMyers flat\tCA\tHumboldt County\tH1\n95568\t6023\tSomes bar\tCA\tHumboldt County\tH1\n95569\t6023\tRedcrest\tCA\tHumboldt County\tH1\n95534\t6023\tCutten\tCA\tHumboldt County\tH1\n95553\t6023\tMiranda\tCA\tHumboldt County\tH1\n92243\t6025\tEl centro\tCA\tImperial County\tH1\n92266\t6025\tPalo verde\tCA\tImperial County\tH1\n92275\t6025\tSalton city\tCA\tImperial County\tH1\n92250\t6025\tHoltville\tCA\tImperial County\tH1\n92231\t6025\tCalexico\tCA\tImperial County\tH1\n92251\t6025\tImperial\tCA\tImperial County\tH1\n92273\t6025\tSeeley\tCA\tImperial County\tH1\n92257\t6025\tNiland\tCA\tImperial County\tH1\n92233\t6025\tCalipatria\tCA\tImperial County\tH1\n92244\t6025\tEl centro\tCA\tImperial County\tH1\n92222\t6025\tBard\tCA\tImperial County\tH1\n92227\t6025\tBrawley\tCA\tImperial County\tH1\n92274\t6025\tThermal\tCA\tImperial County\tH1\n92281\t6025\tWestmorland\tCA\tImperial County\tH1\n92225\t6025\tBlythe\tCA\tImperial County\tH1\n92232\t6025\tCalexico\tCA\tImperial County\tH1\n92259\t6025\tOcotillo\tCA\tImperial County\tH1\n92249\t6025\tHeber\tCA\tImperial County\tH1\n92283\t6025\tWinterhaven\tCA\tImperial County\tH1\n93549\t6027\tOlancha\tCA\tInyo County\tH1\n93526\t6027\tIndependence\tCA\tInyo County\tH1\n92328\t6027\tDeath valley\tCA\tInyo County\tH1\n93515\t6027\tBishop\tCA\tInyo County\tH1\n93545\t6027\tLone pine\tCA\tInyo County\tH1\n93513\t6027\tBig pine\tCA\tInyo County\tH1\n93514\t6027\tBishop\tCA\tInyo County\tH1\n93530\t6027\tKeeler\tCA\tInyo County\tH1\n92384\t6027\tShoshone\tCA\tInyo County\tH1\n93522\t6027\tDarwin\tCA\tInyo County\tH1\n93527\t6027\tInyokern\tCA\tInyo County\tH1\n92389\t6027\tTecopa\tCA\tInyo County\tH1\n93304\t6029\tBakersfield\tCA\tKern County\tH1\n93390\t6029\tBakersfield\tCA\tKern County\tH1\n93560\t6029\tRosamond\tCA\tKern County\tH1\n93504\t6029\tCalifornia city\tCA\tKern County\tH1\n93581\t6029\tTehachapi\tCA\tKern County\tH1\n93385\t6029\tBakersfield\tCA\tKern County\tH1\n93285\t6029\tWofford heights\tCA\tKern County\tH1\n93380\t6029\tBakersfield\tCA\tKern County\tH1\n93205\t6029\tBodfish\tCA\tKern County\tH1\n93243\t6029\tLebec\tCA\tKern County\tH1\n93220\t6029\tEdison\tCA\tKern County\tH1\n93307\t6029\tBakersfield\tCA\tKern County\tH1\n93388\t6029\tBakersfield\tCA\tKern County\tH1\n93215\t6029\tDelano\tCA\tKern County\tH1\n93283\t6029\tWeldon\tCA\tKern County\tH1\n93386\t6029\tBakersfield\tCA\tKern County\tH1\n93556\t6029\tRidgecrest\tCA\tKern County\tH1\n93287\t6029\tWoody\tCA\tKern County\tH1\n93306\t6029\tBakersfield\tCA\tKern County\tH1\n93311\t6029\tBakersfield\tCA\tKern County\tH1\n93555\t6029\tRidgecrest\tCA\tKern County\t
